vi "First Step.vi"(8 "error in (no error)":errorcluster, 11 "Magna Power Scan.lvclass in":refnum<class "Magna Current Scan.lvclass">) -> (0 "error out":errorcluster, 2 "Current Position":dbl, 3 "Magna Power Scan.lvclass out":refnum<class "Magna Current Scan.lvclass">)   [LabVIEW 2017, in "Magna Current Scan.lvclass"]
doc: "(Dynamic) Reset the instrument and prepare to scan. Go to step #0 - the first step. If desired, the scanner may do this in a different way than usual (i.e. by preparing to move a long distance, or reset to home position.)"
uses:
  Magna Current Scan.lvclass
  Instruments/Magna-Power Power Supply/Magna Power.lvclass
  C:/LabVIEW-programs-dev/Instruments/Utility Classes/Scannable/Scannable.lvclass
  Magna Current Scan.lvclass/Magna Current Scan.ctl
  Instruments/Magna-Power Power Supply/Magna Power Constants.vi
  Scanner/Scanner.lvclass
  <vilib>/gmath/NI_Gmath.lvlib
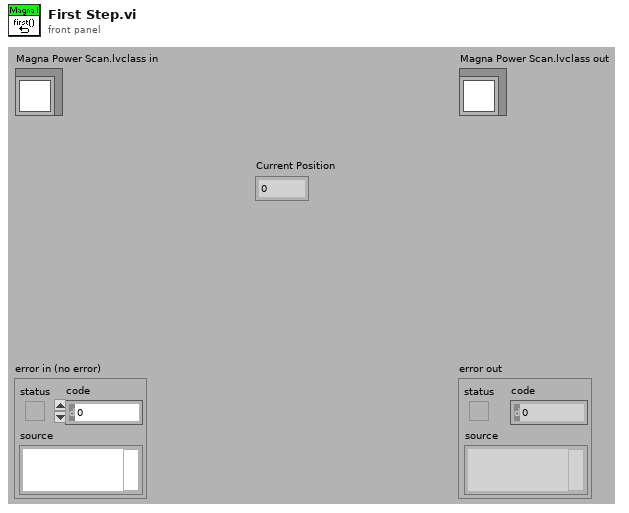
[diagram p1: front panel]
types:
  T1 = cluster{"Magna Current":dbl[], "Magnetic Field":dbl[], "Fluke Voltage":dbl[]}
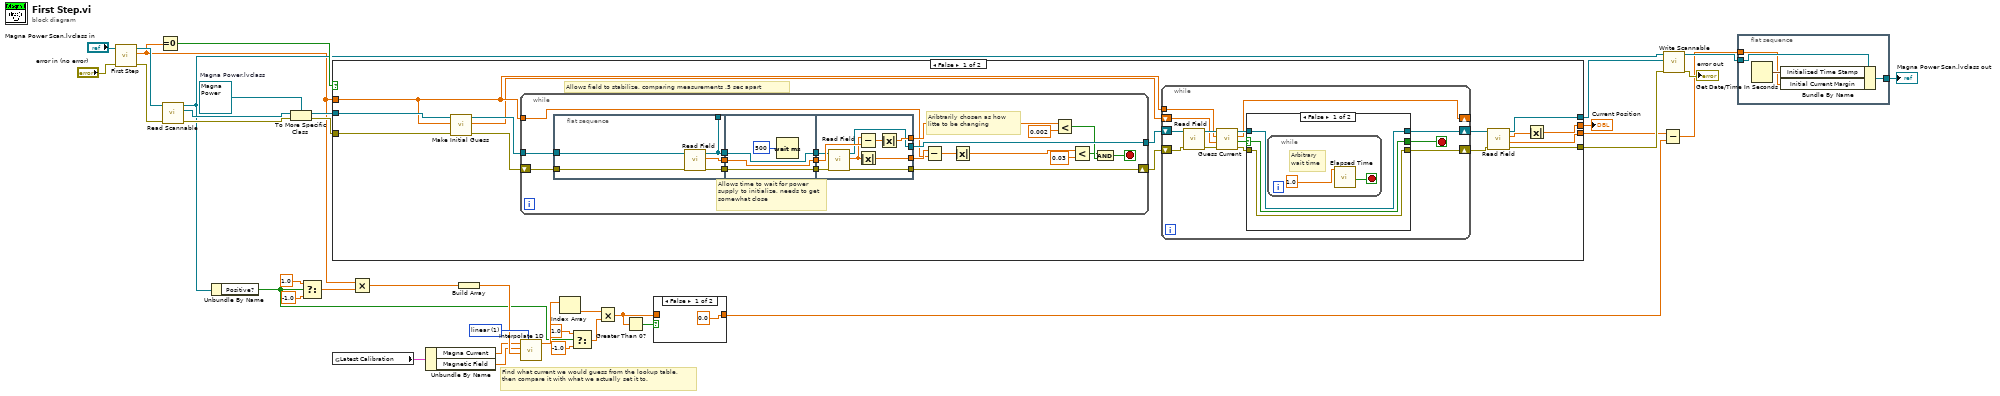
[diagram p0: block diagram]
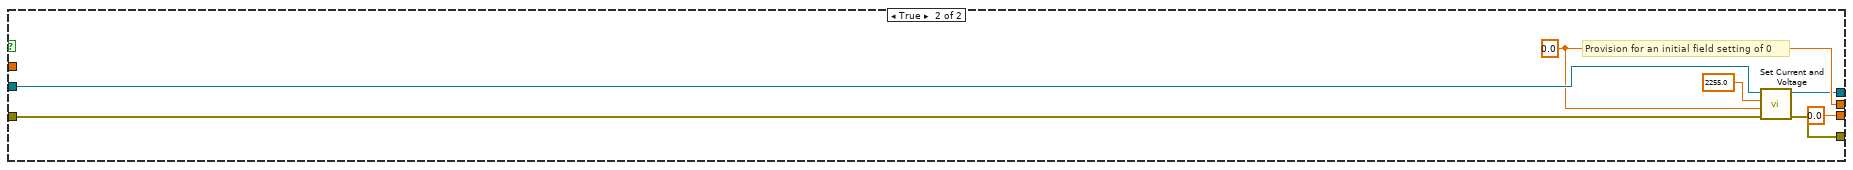
[diagram p4: hidden frame]
diagram:
  w21 = 1 items=["nearest", "linear", "spline", "cubic Hermite", "Lagrange"] ("method")
  w34 = refnum<class "Magna Power.lvclass"> refnum  # Magna Power.lvclass
  # "Find what current we would guess from the lookup table, then compare it with what we actually set it to."
  n1 = call-parent "First Step.vi"("error in (no error)"="error in (no error)", "Scanner.lvclass in"="Magna Power Scan.lvclass in") -> ("error out"=w36:errorcluster, "Current Position"=w4:dbl, "Scanner.lvclass out"=w35:refnum<class "Magna Current Scan.lvclass">)  [unwired: 7 in]
  n2 = Equal To 0?(x=w4) -> (x = 0?=w23:bool)
  n3 = call-dynamic "Read Scannable.vi"("error in (no error)"=w36, "Scanner.lvclass in"=w35) -> ("error out"=w32:errorcluster, "Scannable.lvclass"=w33:refnum<class "Scannable.lvclass">, "Scanner.lvclass out"=w7:refnum<class "Magna Current Scan.lvclass">)  [unwired: 7 in]
  n4 = Unbundle By Name(w7) -> ("Positive?"=w6:bool)
  n5 = To More Specific Class(target class=w34, reference=w33, error in=w32) -> (specific class reference=w30:refnum<class "Magna Power.lvclass">, error out=w31:errorcluster)
  n6 = Select(t=1.0, s=w6, f=-1.0) -> (s? t:f=w8:dbl)
  n7 = case shown="False" w23 {
    tunnel: w31 -> [w49 w119]
    tunnel: w30 -> [w48 w118]
    tunnel: w4 -> [w47 _]
    tunnel: [w45 w115] -> w29
    tunnel: [w42 w116] -> w28
    tunnel: [w43 w114] -> w27
    tunnel: [w40 0.0 ("Numeric")] -> w3
    frame False {
      # "Allows field to stabilize, comparing measurements .5 sec apart"
      n8 = call "Make Initial Guess.vi"("error in (no error)"=w49, "Desired Field"=w47, "Magna Power in"=w48) -> ("error out"=w50:errorcluster, "First guess"=w46:dbl, "Magna Power out"=w51:refnum<class "Magna Power.lvclass">)  [unwired: 6 in]
      n9 = while {
        shift-right: [w88] -> w53
        shift-left: w50 -> [w94]
        tunnel: w51 -> [w86]
        tunnel: [w83] -> w52
        tunnel: w47 -> [w79]
        stop <- w82 stop-if-true
        # "Aribtrarily chosen as how litte to be changing"
        # "Allows time to wait for power supply to initialize, needs to get somewhat close"
        n10 = flat-sequence {
          tunnel: w94 -> [w99]
          tunnel: [w98] -> w92
          tunnel: [w97] -> w90
          tunnel: w86 -> [w96]
          tunnel: [w95] -> w84
          tunnel: [w95] -> _
          tunnel: [w102] -> w93
          tunnel: w92 -> [w102]
          tunnel: [w101] -> w91
          tunnel: w90 -> [w101]
          tunnel: [w100] -> w85
          tunnel: w84 -> [w100]
          tunnel: w93 -> [w112]
          tunnel: w91 -> [w110]
          tunnel: [w109] -> w87
          tunnel: [w108] -> w88
          tunnel: w85 -> [w106]
          tunnel: [w107] -> w83
          tunnel: [w104] -> w80
          frame #0 {
            n11 = call "Read Field.vi"("error in (no error)"=w99, "Magna Power in"=w96) -> ("error out"=w98:errorcluster, "Field (T)"=w97:dbl, "Magna Power out"=w95:refnum<class "Magna Power.lvclass">)  [unwired: 5 in, 2 out]
          }
          frame #1 {
            n12 = Wait (ms)(milliseconds to wait=u32 500) -> ()  [unwired: 1 out]
          }
          frame #2 {
            n13 = call "Read Field.vi"("error in (no error)"=w112, "Magna Power in"=w106) -> ("error out"=w108:errorcluster, "Field (T)"=w105:dbl, "Magna Power out"=w107:refnum<class "Magna Power.lvclass">)  [unwired: 5 in, 2 out]
            n14 = Subtract(x=w105, y=w110) -> (x-y=w111:dbl)
            n15 = Absolute Value(x=w105) -> (abs(x)=w104:dbl)
            n16 = Absolute Value(x=w111) -> (abs(x)=w109:dbl)
          }
        }
        n17 = Subtract(x=w80, y=w79) -> (x-y=w78:dbl)
        n18 = Absolute Value(x=w78) -> (abs(x)=w77:dbl)
        n19 = Less?(x=w87, y=0.002) -> (x < y?=w81:bool)
        n20 = Less?(x=w77, y=0.03) -> (x < y?=w75:bool)
        n21 = And(x=w75, y=w81) -> (x .and. y?=w82:bool)
      }
      n22 = while {
        shift-right: [w62] -> w41
        shift-left: w53 -> [w66]
        shift-right: [w57] -> w44
        shift-left: w52 -> [w61]
        tunnel: w47 -> [w56]
        shift-right: [w54] -> _
        shift-left: w46 -> [w55]
        stop <- w59 stop-if-true
        n23 = call "Read Field.vi"("error in (no error)"=w66, "Magna Power in"=w61) -> ("error out"=w65:errorcluster, "Magna Power out"=w58:refnum<class "Magna Power.lvclass">)  [unwired: 5 in, 3 out]
        n24 = call "Guess Current.vi"("error in (no error)"=w65, "Current guess"=w55, "Desired Field"=w56, "Magna Power in"=w58) -> ("error out"=w63:errorcluster, "Stop?"=w64:bool, "New guess"=w54:dbl, "Magna Power out"=w60:refnum<class "Magna Power.lvclass">)  [unwired: 4 in]
        n25 = case shown="False" w64 {
          selector: w64 -> [w69 w74]
          tunnel: [w69 w74] -> w59
          tunnel: w63 -> [w68 w73]
          tunnel: [w68 w73] -> w62
          tunnel: w60 -> [w67 w72]
          tunnel: [w67 w72] -> w57
          frame False {
            n26 = while {
              stop <- w70 stop-if-true
              # "Arbitrary\nwait time"
              n27 = call "Elapsed Time"("Time Target (s)"=1.0) -> ("Time has Elapsed"=w70:bool)  [unwired: 11 in, 7 out]
            }
          }
          frame True {
          }
        }
      }
      n28 = call "Read Field.vi"("error in (no error)"=w41, "Magna Power in"=w44) -> ("error out"=w42:errorcluster, "Current"=w40:dbl, "Field (T)"=w39:dbl, "Magna Power out"=w43:refnum<class "Magna Power.lvclass">)  [unwired: 5 in, 1 out]
      n29 = Absolute Value(x=w39) -> (abs(x)=w45:dbl)
    }
    frame True {
      w115 = 0.0 ("Current Limit")
      # "Provision for an initial field setting of 0"
      n30 = call "Set Current and Voltage.vi"("error in (no error)"=w119, "Current Limit"=w115, "Voltage Limit"=2255.0, "Magna Power in"=w118) -> ("error out"=w116:errorcluster, "Magna Power out"=w114:refnum<class "Magna Power.lvclass">)  [unwired: 6 in]
    }
  }
  "Current Position" <- w29
  n31 = global read "Magna Power Constants.vi" "Latest Calibration"() -> (w22:T1)
  n32 = Multiply(x=w4, y=w8) -> (x*y=w5:dbl)
  n33 = Unbundle By Name(w22) -> ("Magna Current"=w17:dbl[], "Magnetic Field"=w18:dbl[])
  n34 = Build Array(w5) -> (w20:dbl[])
  n35 = call <vilib>:"Interpolate 1D.vi"("method"=w21, "xi"=w20, "X"=w18, "Y"=w17) -> ("yi"=w19:dbl[])  [unwired: 5 in, 2 out]
  n36 = Index Array(array=w19) -> (element=w13:dbl)  [unwired: 1 in]
  n37 = Select(t=1.0, s=w6, f=-1.0) -> (s? t:f=w12:dbl)
  n38 = Multiply(x=w13, y=w12) -> (x*y=w11:dbl)
  n39 = Greater Than 0?(x=w11) -> (x > 0?=w16:bool)
  n40 = case shown="False" w16 {
    tunnel: [0.0 ("Numeric") w121] -> w2
    tunnel: w11 -> [_ w121]
    frame False {
    }
    frame True {
    }
  }
  n41 = Subtract(x=w3, y=w2) -> (x-y=w1:dbl)
  n42 = call-dynamic "Write Scannable.vi"("error in (no error)"=w28, "Scannable.lvclass"=w27, "Scanner.lvclass in"=w7) -> ("error out"=→"error out":errorcluster, "Scanner.lvclass out"=w25:refnum<class "Magna Current Scan.lvclass">)  [unwired: 7 in]
  n43 = flat-sequence {
    tunnel: w25 -> [w124]
    tunnel: [w123] -> w24
    tunnel: w1 -> [w122]
    frame #0 {
      n44 = Get Date/Time In Seconds() -> (seconds since 1Jan1904=w125:timestamp)
      n45 = Bundle By Name(cluster=w124, "Initialized Time Stamp"=w125, "Initial Current Margin"=w122) -> (w123:refnum<class "Magna Current Scan.lvclass">)
    }
  }
  "Magna Power Scan.lvclass out" <- w24
